vi "Kapitza Main.vi"   [LabVIEW 2018]
doc: "This template is for the Queued Message Handler design pattern.\n\nThe Event Handling Loop generates messages based on user interface actions.\n\nThe Message Handling Loop processes messages generated by the Event Handling Loop, or by other messages. The messages are string values, so new messages can be added easily to the Message Cases case structure in the Message Handling Loop. Each message cluster can also provide an optional value for Message Data, which is a variant that can be converted to whatever message-specific data is required."
uses:
  controls/Kapitza UI Data.ctl
  support/Message Queue/Kapitza Message Queue.lvlib
  <vilib>/Utility/error.llb/Error Cluster From Error Code.vi
  support/User Event - Stop/Kapitza User Event - Stop.lvlib
  support/Message Queue/Enqueue Message (Single).vi
  <vilib>/ErrorRing/Error Ring.xnode
panel:
  # "These controls have associated \"Value Changed\" events configured in the Event Structure on the diagram.\n\nReplace them (and reconfigure the Event Structure) with the controls you need for your application."
  # "This template is for the Queued Message Handler design pattern.\n\nSee the block diagram for more information on how to use this template."
types:
  T1 = typedef "Kapitza UI Data.ctl" = cluster{"Boolean <Replace Me>":bool, "String <Replace Me>":string, "Numeric <Replace Me>":dbl, "Do Something Ref":refnum<vi>, "Do Something Else Ref":refnum<vi>, "Data Display Ref":refnum<vi>, "Exit Button Ref":refnum<vi>}
  T2 = typedef "Kapitza Message Queue.lvlib/All Message Queues.ctl" = cluster{"UI":refnum<queue>}
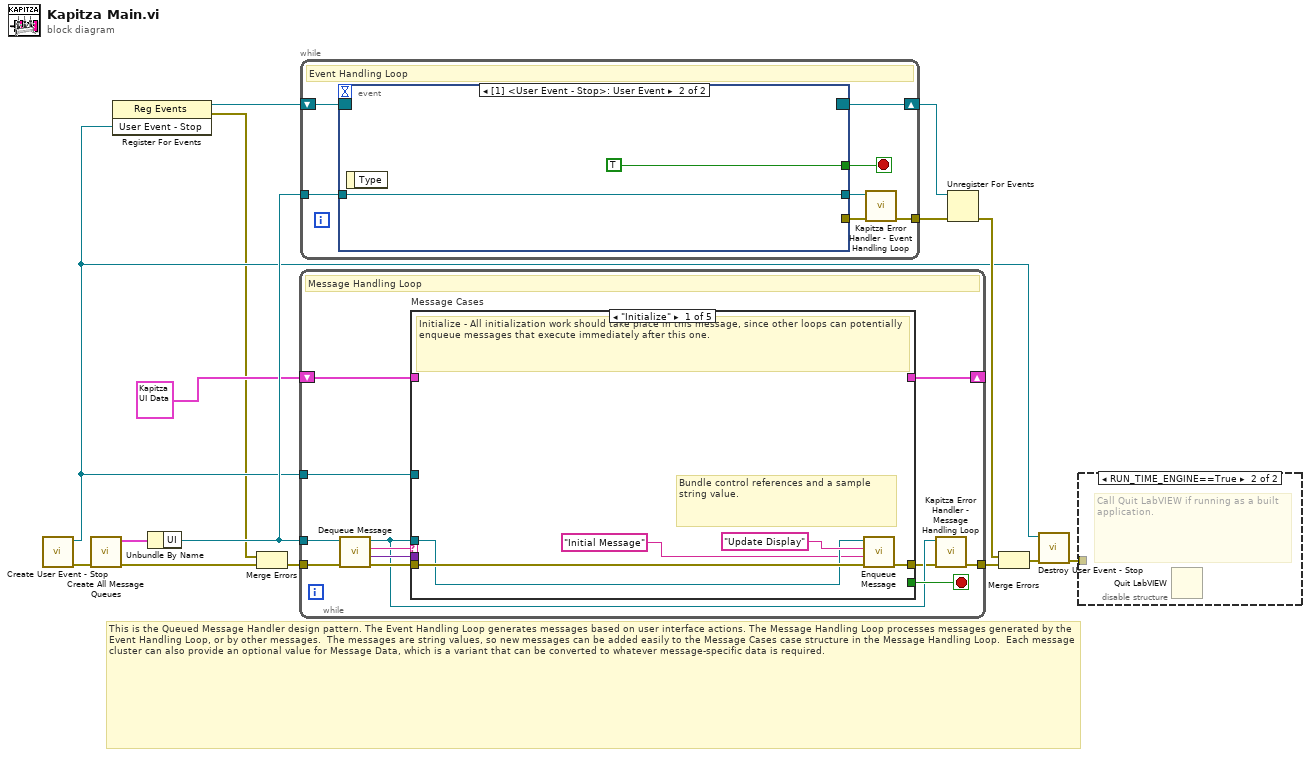
[diagram p0: block diagram]
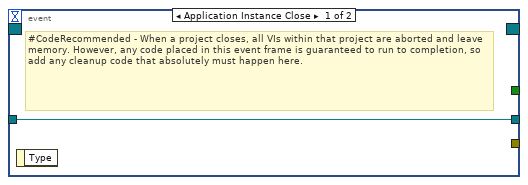
[diagram p3: hidden frame]
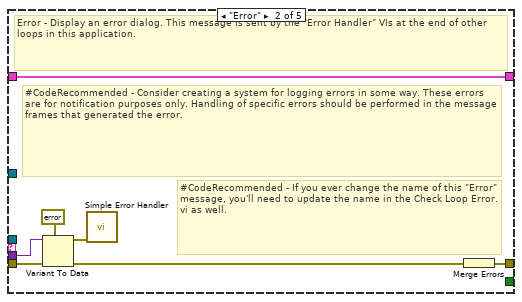
[diagram p4: hidden frame]
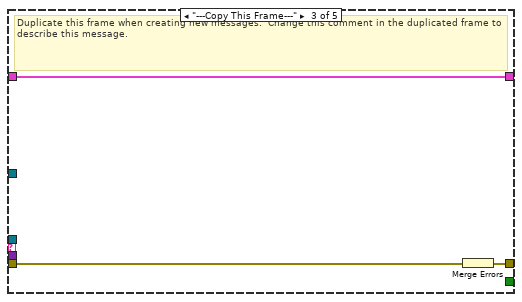
[diagram p5: hidden frame]
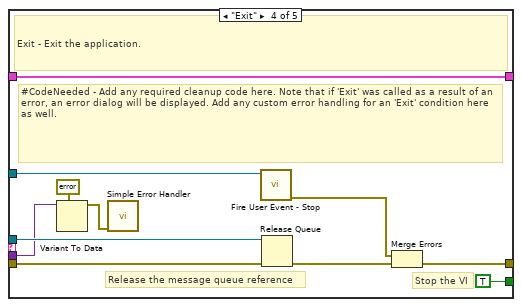
[diagram p6: hidden frame]
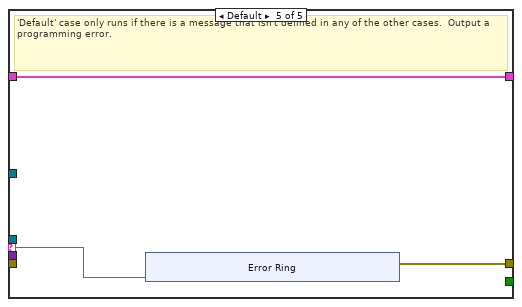
[diagram p7: hidden frame]
diagram:
  # "This is the Queued Message Handler design pattern. The Event Handling Loop generates messages based on user interface actions. The Message Handling Loop processes messages generated by the Event Handling Loop, or by other messages.  The messages are string values, so new messages can be added easily to the Message Cases case structure in the Message Handling Loop.  Each message cluster can also provide an optional value for Message Data, which is a variant that can be converted to whatever message-specific data is required."
  n1 = call "Create User Event - Stop.vi"() -> ("error out"=w11:errorcluster, "User Event - Stop"=w3:refnum<user-event>)  [unwired: 10 in]
  n2 = call "Create All Message Queues.vi"("error in (no error)"=w11) -> ("error out"=w15:errorcluster, "Message Queues out"=w14:T2)  [unwired: 9 in]
  n3 = register-events(w3) -> (reference out=w4:refnum<event-registration>, error out=w1:errorcluster)  [unwired: 2 in]
  n4 = Unbundle By Name(w14) -> ("UI"=w12:refnum<queue>)
  n5 = Merge Errors(w1, w15) -> (w2:errorcluster)
  n6 = while {
    tunnel: w12 -> [w19]
    shift-right: [w26] -> _
    shift-left: T1 {"Boolean <Replace Me>"=FALSE, "String <Replace Me>"="", "Numeric <Replace Me>"=0.0, "Do Something Ref"=refnum, "Do Something Else Ref"=refnum, "Data Display Ref"=refnum, "Exit Button Ref"=refnum} ("Data Cluster") -> [w27]
    tunnel: w3 -> [w24]
    tunnel: w2 -> [w23]
    tunnel: [w17] -> w13
    stop <- w25 stop-if-true
    # "Message Handling Loop"
    n7 = call "Dequeue Message.vi"("error in (no error)"=w23, "Message Queue"=w19) -> ("error out"=w22:errorcluster, "Message Data"=w20:variant, "Message"=w21:string, "dup Message Queue"=w18:refnum<queue>)  [unwired: 6 in]
    n8 = case "Message Cases" shown="\"Initialize\"" w21 {
      selector: w21 -> [_ _ _ _ w54]
      tunnel: w18 -> [w29 _ _ w53 _]
      tunnel: w22 -> [w31 w39 w42 w46 _]
      tunnel: [w32 w33 w40 w49 w55] -> w16
      tunnel: w27 -> [_ w38 w41 w52 w56]
      tunnel: [_ w38 w41 w52 w56] -> w26
      tunnel: [_ _ _ TRUE _] -> w25
      tunnel: w20 -> [_ w37 _ w43 _]
      tunnel: w24 -> [_ _ _ w48 _]
      frame "Initialize" {
        # "Bundle control references and a sample string value."
        # "Initialize - All initialization work should take place in this message, since other loops can potentially enqueue messages that execute immediately after this one."
        n9 = call-poly "Enqueue Message.vi"("error in (no error)"=w31, "Message Data"="Initial Message" ("Initial Message"), "Message"="Update Display", "Message Queue"=w29) -> ("error out"=w32:errorcluster)  [unwired: 6 in, 1 out]
      }
      frame "Error" {
        # "#CodeRecommended - If you ever change the name of this \"Error\" message, you'll need to update the name in the Check Loop Error.vi as well."
        # "#CodeRecommended - Consider creating a system for logging errors in some way. These errors are for notification purposes only. Handling of specific errors should be performed in the message frames that generated the error."
        # "Error - Display an error dialog. This message is sent by the \"Error Handler\" VIs at the end of other loops in this application."
        n10 = Variant To Data(error in=w39, type=errorcluster {"status"=FALSE, "code"=0, "source"=""} ("error constant"), Variant=w37) -> (data=w35:errorcluster, error out=w34:errorcluster)
        n11 = call <vilib>:"Simple Error Handler.vi"("error in (no error)"=w35) -> ()  [unwired: 4 in, 5 out]
        n12 = Merge Errors(w34) -> (w33:errorcluster)
      }
      frame "---Copy This Frame---" {
        # "Duplicate this frame when creating new messages.  Change this comment in the duplicated frame to describe this message."
        n13 = Merge Errors(w42) -> (w40:errorcluster)
      }
      frame "Exit" {
        # "Stop the VI"
        # "Release the message queue reference"
        # "#CodeNeeded - Add any required cleanup code here. Note that if 'Exit' was called as a result of an error, an error dialog will be displayed. Add any custom error handling for an 'Exit' condition here as well."
        # "Exit - Exit the application."
        n14 = Variant To Data(type=errorcluster {"status"=FALSE, "code"=0, "source"=""} ("error constant"), Variant=w43) -> (data=w44:errorcluster)  [unwired: 1 in, 1 out]
        n15 = call <vilib>:"Simple Error Handler.vi"("error in (no error)"=w44) -> ()  [unwired: 4 in, 5 out]
        n16 = call "Fire User Event - Stop.vi"("User Event - Stop"=w48) -> ("error out"=w47:errorcluster)  [unwired: 10 in]
        n17 = Release Queue(queue=w53, error in (no error)=w46) -> (error out=w50:errorcluster)  [unwired: 1 in, 2 out]
        n18 = Merge Errors(w47, w50) -> (w49:errorcluster)
      }
      frame Default {
        # "'Default' case only runs if there is a message that isn't defined in any of the other cases.  Output a programming error."
        n19 = xnode "Error Ring"("parameter 0"=w54) -> ("error out"=w55:errorcluster)
      }
    }
    n20 = call "Kapitza Error Handler - Message Handling Loop.vi"("error in (no error)"=w16, "Message Queue"=w18) -> ("dup error in"=w17:errorcluster)  [unwired: 8 in, 1 out]
  }
  n21 = while {
    tunnel: w12 -> [w70]
    shift-right: [w68] -> w8
    shift-left: w4 -> [w69]
    tunnel: [w64] -> w5
    stop <- w66 stop-if-true
    # "Event Handling Loop"
    n22 = event shown="[1] <User Event - Stop>: User Event" {
      selector: w69 -> [_ _]
      dyn-events: [_ _] -> w68
      timeout: _ -> [_ _]
      tunnel: [_ TRUE ("Discard?")] -> w66
      tunnel: w70 -> [w71 w73]
      tunnel: [_ _] -> w67
      tunnel: [w71 w73] -> w65
      event Application Instance Close {
        # "#CodeRecommended - When a project closes, all VIs within that project are aborted and leave memory. However, any code placed in this event frame is guaranteed to run to completion, so add any cleanup code that absolutely must happen here."
        n23 = event-data() -> ()  [unwired: 1 in, 1 out]
      }
      event User Event {
        n24 = event-data() -> ()  [unwired: 1 in, 1 out]
      }
    }
    n25 = call "Kapitza Error Handler - Event Handling Loop.vi"("error in (no error)"=w67, "Message Queue"=w65) -> ("dup error in"=w64:errorcluster)  [unwired: 8 in, 1 out]
  }
  n26 = Unregister For Events(event registration refnum=w8, error in=w5) -> (error out=w9:errorcluster)
  n27 = Merge Errors(w9, w13) -> (w10:errorcluster)
  n28 = call "Destroy User Event - Stop.vi"("error in (no error)"=w10, "User Event - Stop"=w3) -> ("error out"=w6:errorcluster)  [unwired: 9 in]
  n29 = disable-structure shown="RUN_TIME_ENGINE==True" {
    disable-tunnel: w6 -> [_ _]
    frame condition #0 (active) {
    }
    frame condition #1 {
      # "Call Quit LabVIEW if running as a built application."
      n30 = Quit LabVIEW() -> ()  [unwired: 1 in]
    }
  }
